vi "ConvertTo(multiloopErrorHandler).vi"(8 "error in":errorcluster, 9 "Message Payload":variant) -> (0 "error out":errorcluster, 1 "Message Payload error":errorcluster, 2 "Handle Loop Que":bool)   [LabVIEW 2019]
doc: "Convert variant to error cluster and flush buffer TF for receiving an erro message in a multiloop state machine\n\nBolder Software LLC"
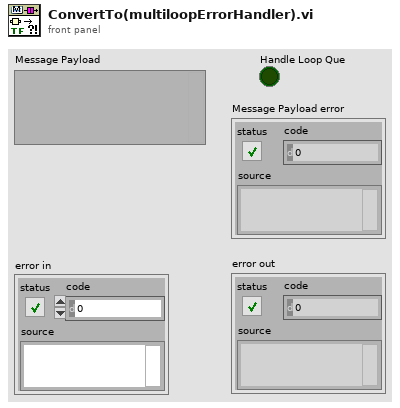
[diagram p1: front panel]
types:
  T1 = cluster{"Handle Loop Que":bool, "error":errorcluster}
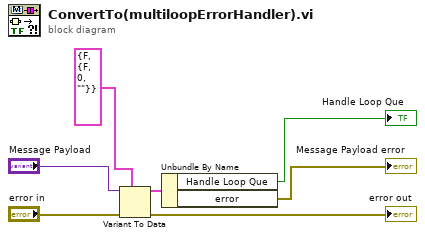
[diagram p0: block diagram]
diagram:
  n1 = Variant To Data(error in="error in", type=T1 {"Handle Loop Que"=FALSE, "error"={"status"=FALSE, "code"=0, "source"=""}} ("Message Payload  multiloopError cluster"), Variant="Message Payload") -> (data=w3:T1, error out=→"error out":errorcluster)
  n2 = Unbundle By Name(w3) -> ("Handle Loop Que"=→"Handle Loop Que":bool, "error"=→"Message Payload error":errorcluster)
